vi "DFD M-Band Filter Bank Reconstruction with State (Array).vi"(6 "state in":cluster{"state ":dbl[]}[](array[cluster]), 8 "error in (no error)":errorcluster, 9 "init? (F)":bool, 10 "synthesis bank":T1={"mBank_Filters"=[], " mBank_#Bands"=2, "mBank_ProcMethod"=enum."General", "mBank_Coeffs"=[], "mBank_Gain"=1.0, "mBank_Type"=0} {"mBank_Type" items=["Uniform", "Non-Uniform"]; "mBank_Filters"."mMRate_SumWl" min=1 max=32 step=1; "mBank_Filters"."mMRate_InputIwl" min=1 max=32 step=1; "mBank_Filters"."mMRate_GainWl" min=1 max=32 step=1; "mBank_Filters"."mMRate_OutputWl" min=1 max=32 step=1; "mBank_Filters"."mMRate_InputWl" min=1 max=32 step=1; "mBank_Filters"."mMRate_CoefWl" min=1 max=32 step=1; "mBank_Filters"."mMRate_Mode" items=["Default"=-1, "No Rate Change"=0, "Interpolation"=1, "Decimation"=2, "Interpolated"=3, "Rational"=4]}, 11 "M bands":dbl[][](array[numeric])) -> (0 "error out":errorcluster, 3 "y":dbl[](array[numeric]), 4 "state out":cluster{"state ":dbl[]}[](array[cluster]))   [LabVIEW 2017, in "NI_DigFilter_FilterBank.lvlib"]
doc: "Reconstructs signal from M-channel sequences <B>x</B> using an M-band synthesis bank specified by <B>synthesis bank</B>. You must specify the most recent internal input states <B>state in</B> to get the correct output. \n\n<B>state out</B> contains the most recent internal output states, which can be used as <B>state in</B> for next call to this VI if you want to process the data continuously.\n\nYou can call the VIs in <B>Filter Bank Design</B> sub-palette to design a filter bank."
uses:
  <vilib>/addons/Digital Filter Design/NI_DigFilter_FilterBank.lvlib
  <vilib>/addons/Digital Filter Design/FilterBank.llb/Object/DFD Bank Obj.ctl
  <vilib>/addons/Digital Filter Design/_Objects.llb/DFD Multirate Filter Obj.ctl
  <vilib>/addons/Digital Filter Design/_Objects.llb/DFD Multirate Mode.ctl
  <vilib>/addons/Digital Filter Design/_Objects.llb/DFD Coef Norm Type.ctl
  <vilib>/addons/Digital Filter Design/_Objects.llb/DFD Round-off Mode.ctl
  <vilib>/addons/Digital Filter Design/_Objects.llb/DFD FXP MRate Multiply Mode.ctl
  <vilib>/addons/Digital Filter Design/FilterBank.llb/Object/DFD Filter Bank Processing Method.ctl
  <vilib>/addons/Digital Filter Design/FilterBank.llb/Object/DFD Filter Bank Type.ctl
  <vilib>/addons/Digital Filter Design/NI_DigFilterLicensed.lvlib
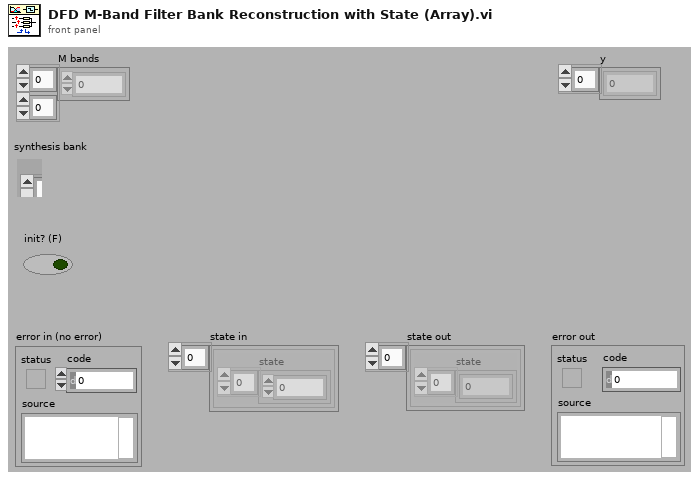
[diagram p1: front panel]
types:
  T1 = typedef "NI_DigFilter_FilterBank.lvlib/DFD Bank Obj.ctl" = cluster{"mBank_Filters":T2[], " mBank_#Bands":i32, "mBank_ProcMethod":T7, "mBank_Coeffs":dbl[], "mBank_Gain":dbl, "mBank_Type":T8}
  T2 = typedef "NI_DigFilterLicensed.lvlib/DFD Multirate Filter Obj.ctl" = cluster{"mMRate_Structure":enum16{"CIC", "FIR", "IIR", "Lattice"}, "mMRate_Mode":T3, "mMRate_Factor":i32, "mMRate_FIRParams":cluster{"mMRate_FIR_H":dbl[], "mMRate_FIR_IsNyquist?":bool, "mMRate_FIR_IsSymmetric?":bool}, "mMRate_CICParams":cluster{"mMRate_CIC_#Stage":i32, "mMRate_CIC_Lag":i32, "mMRate_CIC_Type":enum16{"Lowpass", "Highpass"}}, "mMRate_Order":i32, "mMRate_Version":string, "mMRate_Comments":string, "mMRate_RationalFactor":cluster{"mMRate_L":i32, "mMRate_M":i32}, "mMRate_Fs":dbl, "mMRate_Quantized?":bool, "mMRate_QFilterGain":dbl, "mMRate_CoefWl":i16, "mMRate_Scaling":cluster{"mMRate_ScaleByPowerOf2?":bool, "mMRate_ScaleType":T4}, "mMRate_InputWl":i16, "mMRate_OutputWl":i16, "mMRate_OutputMode":T5, "mMRate_MultMode":T6, "mMRate_BitPruning":bool, "mMRate_GainWl":i16, "mMRate_OutputFwl":i16, "mMRate_SumIwl":i16, "mMRate_InputIwl ":i16, "mMRate_SumWl":i16, "mMRate_CoefIwl":i16}
  T3 = typedef "NI_DigFilterLicensed.lvlib/DFD Multirate Mode.ctl" = i16
  T4 = typedef "NI_DigFilterLicensed.lvlib/DFD Coef Norm Type.ctl" = enum16{"No Norm", "Time Domain 1-Norm", "Time Domain 2-Norm", "Time Domain Inf-Norm"}
  T5 = typedef "NI_DigFilterLicensed.lvlib/DFD Round-off Mode.ctl" = enum16{"Nearest", "Truncation"}
  T6 = typedef "NI_DigFilterLicensed.lvlib/DFD FXP MRate Multiply Mode.ctl" = enum16{"Truncated", "Full"}
  T7 = typedef "NI_DigFilter_FilterBank.lvlib/DFD Filter Bank Processing Method.ctl" = enum16{"General", "2-Band QMF Lattice", "Cosine-Modulated"}
  T8 = typedef "NI_DigFilter_FilterBank.lvlib/DFD Filter Bank Type.ctl" = u16
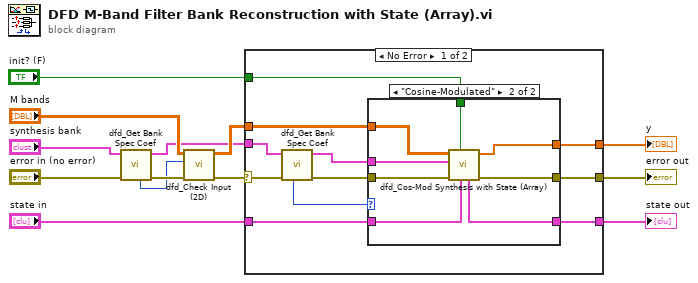
[diagram p0: block diagram]
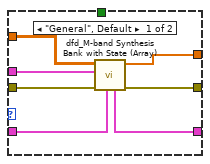
[diagram p2: hidden frame]
diagram:
  n1 = call <vilib>:"dfd_Get Bank Spec Coef.vi"("error in (no error)"="error in (no error)", "bank in"="synthesis bank") -> ("error out"=w7:errorcluster, "bank out"=w3:T1, "number of bands"=w2:i32)  [unwired: 4 in, 3 out]
  n2 = call <vilib>:"dfd_Check Input (2D).vi"("error in (no error)"=w7, "number of bands"=w2, "x"="M bands") -> ("error out"=w6:errorcluster, "dup x"=w4:dbl[][])  [unwired: 7 in]
  n3 = case shown="No Error" w6 {
    selector: w6 -> [w20 w40]
    tunnel: [w23 _] -> w13
    tunnel: [w22 w40] -> w12
    tunnel: [w15 _] -> w11
    tunnel: "state in" -> [w24 _]
    tunnel: w3 -> [w21 _]
    tunnel: w4 -> [w17 _]
    tunnel: "init? (F)" -> [w14 _]
    frame No Error {
      n4 = call <vilib>:"dfd_Get Bank Spec Coef.vi"("error in (no error)"=w20, "bank in"=w21) -> ("error out"=w16:errorcluster, "bank out"=w18:T1, "processing method"=w19:T7)  [unwired: 4 in, 3 out]
      n5 = case shown="\"Cosine-Modulated\"" w19 {
        tunnel: [w27 w37] -> w23
        tunnel: w17 -> [w31 w39]
        tunnel: [w28 w35] -> w22
        tunnel: [w29 w33] -> w15
        tunnel: w24 -> [w30 w36]
        tunnel: w18 -> [w25 w38]
        tunnel: w16 -> [w26 w34]
        tunnel: w14 -> [_ w32]
        frame "General", Default {
          n6 = call <vilib>:"dfd_M-band Synthesis Bank with State (Array).vi"("state in"=w30, "error in (no error)"=w26, "filter bank in"=w25, "x"=w31) -> ("error out"=w28:errorcluster, "y"=w27:dbl[], "state out"=w29:cluster{"state ":dbl[]}[])  [unwired: 5 in]
        }
        frame "Cosine-Modulated" {
          n7 = call <vilib>:"dfd_Cos-Mod Synthesis with State (Array).vi"("state in"=w36, "init?"=w32, "error in (no error)"=w34, "synthesis bank"=w38, "x"=w39) -> ("error out"=w35:errorcluster, "y"=w37:dbl[], "state out"=w33:cluster{"state ":dbl[]}[])  [unwired: 4 in]
        }
      }
    }
    frame Error {
    }
  }
  "error out" <- w12
  "y" <- w13
  "state out" <- w11
